vi "Initialize Data Ref.vi"(8 "error in (no error)":errorcluster, 10 "Data Ref":T1, 11 "VeriStand Data Sharing Framework in":refnum<class "VeriStand DSF.lvclass">) -> (0 "error out":errorcluster, 3 "VeriStand Data Sharing Framework out":refnum<class "VeriStand DSF.lvclass">)   [LabVIEW 2017, in "DSF Engine.lvlib" / "VeriStand DSF.lvclass"]
uses:
  VeriStand DSF.lvclass
  <vilib>/NI Veristand/Custom Device API/Data Table Ref.ctl
  DSF Core.lvlibp/Classes/Framework/Framework.lvclass
  C:/Git/DSF/VeriStand/Data Sharing Custom Device/Source/DSF Core.lvlibp/Classes/Framework/Framework.lvclass
  <vilib>/NI Veristand/Custom Device API/Custom Device API.lvlib
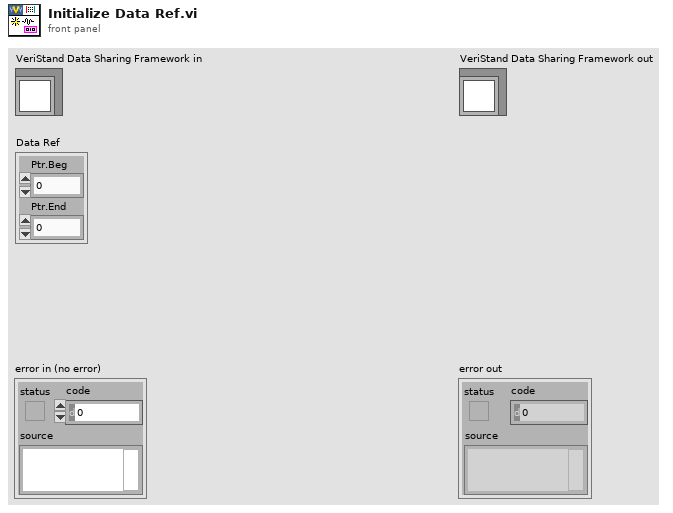
[diagram p1: front panel]
types:
  T1 = typedef "Custom Device API.lvlib/Data Table Ref.ctl" = cluster{"Ptr.Beg":u64, "Ptr.End":u64}
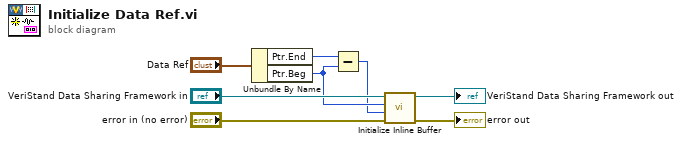
[diagram p0: block diagram]
diagram:
  n1 = Unbundle By Name("Data Ref") -> ("Ptr.End"=w4:u64, "Ptr.Beg"=w3:u64)
  n2 = Subtract(x=w4, y=w3) -> (x-y=w2:u64)
  n3 = call "Initialize Inline Buffer.vi"("error in (no error)"="error in (no error)", "size"=w2, "address"=w3, "Framework in"="VeriStand Data Sharing Framework in") -> ("error out"=→"error out":errorcluster, "Framework out"=→"VeriStand Data Sharing Framework out":refnum<class "VeriStand DSF.lvclass">)  [unwired: 6 in]
